vi "NISE.Open Device Command.vi"(0 "SLSC Interface in":refnum<class "SLSC Interface.lvclass">, 5 "device":refnum<k21>="$DefaultDevices", 7 "command in":refnum<k21>, 11 "error in (no error)":errorcluster) -> (4 "SLSC Interface out":refnum<class "SLSC Interface.lvclass">, 8 "command out":refnum<k21>, 15 "error out":errorcluster)   [LabVIEW 2016, in "SLSC Interface.lvclass"]
uses:
  SLSC Interface.lvclass
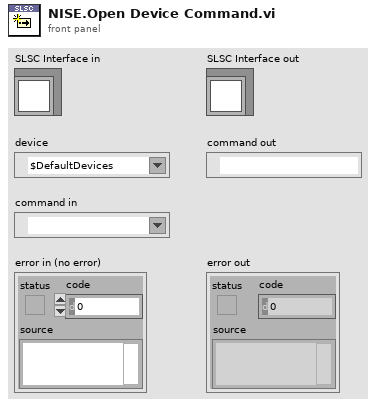
[diagram p1: front panel]
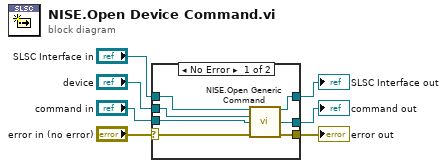
[diagram p0: block diagram]
diagram:
  n1 = case shown="No Error" "error in (no error)" {
    selector: "error in (no error)" -> [w12 w16]
    tunnel: [w11 w16] -> w6
    tunnel: [w13 w15] -> w4
    tunnel: "SLSC Interface in" -> [w14 w15]
    tunnel: "device" -> [w10 _]
    tunnel: "command in" -> [w9 _]
    tunnel: [w8 _] -> w1
    frame No Error {
      n2 = call "NISE.Open Generic Command.vi"("SLSC Interface in"=w14, "resource"=w10, "command in"=w9, "error in (no error)"=w12) -> ("SLSC Interface out"=w13:refnum<class "SLSC Interface.lvclass">, "command out"=w8:refnum<k21>, "error out"=w11:errorcluster)  [unwired: 9 in]
    }
    frame Error {
    }
  }
  "error out" <- w6
  "SLSC Interface out" <- w4
  "command out" <- w1
